vi "GetProperties.vi"(8 "error in":errorcluster, 11 "WaveformGraph in":refnum<class "WaveformGraph.lvclass">) -> (0 "error out":errorcluster, 3 "WaveformGraph out":refnum<class "WaveformGraph.lvclass">)   [LabVIEW 2014, in "Raspberry Pi Compatible Compiler for LabVIEW.lvlib" / "WaveformGraph.lvclass"]
uses:
  WaveformGraph.lvclass
  WaveformGraph.lvclass/WaveformGraph.ctl
  GraphChart/GraphChart.lvclass
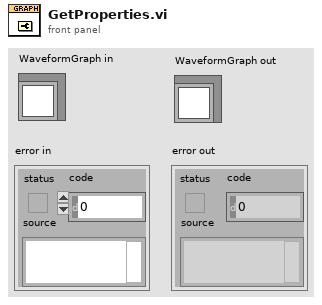
[diagram p1: front panel]
types:
  T1 = typedef "LVPositionTypeDef.ctl" = cluster{"Left":i32, "Top":i32}
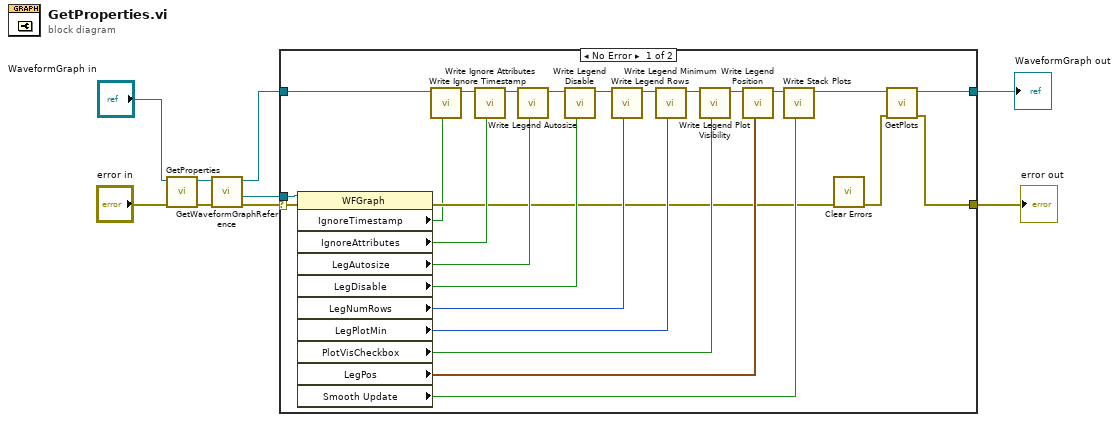
[diagram p0: block diagram]
diagram:
  n1 = call-parent "GetProperties.vi"("error in"="error in", "GraphChart in"="WaveformGraph in") -> ("error out"=w6:errorcluster, "GraphChart out"=w7:refnum<class "WaveformGraph.lvclass">)  [unwired: 8 in]
  n2 = call "GetWaveformGraphReference.vi"("error in"=w6, "WFGraph in"=w7) -> ("error out"=w5:errorcluster, "WFGraph reference"=w4:refnum<vi>, "WFGraph out"=w3:refnum<class "WaveformGraph.lvclass">)  [unwired: 7 in]
  n3 = case shown="No Error" w5 {
    selector: w5 -> [w33 w35]
    tunnel: w4 -> [w34 _]
    tunnel: w3 -> [w11 w36]
    tunnel: [w17 w36] -> w2
    tunnel: [w15 w35] -> w1
    frame No Error {
      n4 = property class="WFGraph"(reference=w34, error in=w33) -> (error out=w14:errorcluster, "IgnoreTimestamp"=w10:bool, "IgnoreAttributes"=w28:bool, "LegAutosize"=w27:bool, "LegDisable"=w26:bool, "LegNumRows"=w24:u32, "LegPlotMin"=w23:u32, "PlotVisCheckbox"=w21:bool, "LegPos"=w20:T1, "Smooth Update"=w19:bool)  [unwired: 1 out]
      n5 = call "Write Ignore Timestamp.vi"("Ignore Timestamp"=w10, "WaveformGraph in"=w11) -> ("WaveformGraph out"=w12:refnum<class "WaveformGraph.lvclass">)  [unwired: 7 in]
      n6 = call "Write Ignore Attributes.vi"("Ignore Attributes"=w28, "WaveformChart in"=w12) -> ("WaveformChart out"=w32:refnum<class "WaveformGraph.lvclass">)  [unwired: 7 in]
      n7 = call "Write Legend Autosize.vi"("Legend Autosize"=w27, "WaveformChart in"=w32) -> ("WaveformChart out"=w31:refnum<class "WaveformGraph.lvclass">)  [unwired: 7 in]
      n8 = call "Write Legend Disable.vi"("Legend Disable"=w26, "WaveformChart in"=w31) -> ("WaveformChart out"=w25:refnum<class "WaveformGraph.lvclass">)  [unwired: 7 in]
      n9 = call "Write Legend Rows.vi"("Legend Rows"=w24, "WaveformChart in"=w25) -> ("WaveformChart out"=w22:refnum<class "WaveformGraph.lvclass">)  [unwired: 7 in]
      n10 = call "Write Legend Minimum.vi"("Legend Minimum"=w23, "WaveformChart in"=w22) -> ("WaveformChart out"=w30:refnum<class "WaveformGraph.lvclass">)  [unwired: 7 in]
      n11 = call "Write Legend Plot Visibility.vi"("Legend Plot Visibility"=w21, "WaveformChart in"=w30) -> ("WaveformChart out"=w29:refnum<class "WaveformGraph.lvclass">)  [unwired: 7 in]
      n12 = call "Write Legend Position.vi"("Legend Position"=w20, "WaveformChart in"=w29) -> ("WaveformChart out"=w18:refnum<class "WaveformGraph.lvclass">)  [unwired: 7 in]
      n13 = call "Write Stack Plots.vi"("Stack Plots"=w19, "WaveformChart in"=w18) -> ("WaveformChart out"=w13:refnum<class "WaveformGraph.lvclass">)  [unwired: 7 in]
      n14 = call <vilib>:"Clear Errors.vi"("error in (no error)"=w14) -> ("error out"=w16:errorcluster)  [unwired: 5 in, 1 out]
      n15 = call "GetPlots.vi"("error in"=w16, "WaveformChart in"=w13) -> ("error out"=w15:errorcluster, "WaveformChart out"=w17:refnum<class "WaveformGraph.lvclass">)  [unwired: 8 in]
    }
    frame Error {
    }
  }
  "error out" <- w1
  "WaveformGraph out" <- w2
